vi "Merge Error Conditional.vi"(7 "Merge Error? (true)":bool=TRUE, 10 "Error To Merge":errorcluster, 11 "Original Error Wire":errorcluster) -> (3 "Error Out":errorcluster)   [LabVIEW 2014, in "i3-sse-server.lvlib"]
uses:
  i3-sse-server.lvlib
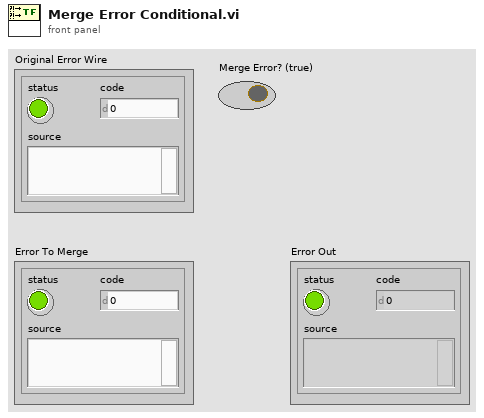
[diagram p1: front panel]
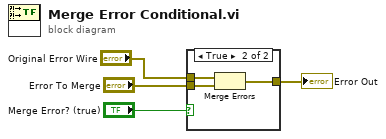
[diagram p0: block diagram]
diagram:
  n1 = case shown="True" "Merge Error? (true)" {
    tunnel: "Original Error Wire" -> [w5 w8]
    tunnel: "Error To Merge" -> [_ w7]
    tunnel: [w5 w6] -> w1
    frame False {
    }
    frame True {
      n2 = Merge Errors(w8, w7) -> (w6:errorcluster)
    }
  }
  "Error Out" <- w1
